vi "PH_gentec_P-Link.set Head Attenuator.vi"(0 "i ref in":refnum<vi>, 2 "VISA resource in":refnum<visa-resource-name>, 5 "error in":errorcluster) -> (11 "Timeout":bool, 13 "Data read":string[](array[string]), 14 "i ref out":refnum<vi>, 16 "VISA resource out":refnum<visa-resource-name>, 17 "Error":bool, 19 "error out":errorcluster)   [LabVIEW 2014, in "PH_gentec_P-Link.lvlib"]
doc: "This VI writes wanted Settings to the Device and checks the result."
uses:
  PH_gentec_P-Link.lvlib
  instr.lib/Gentec-M-Link/gentec-M-Link - Driver.lvlib
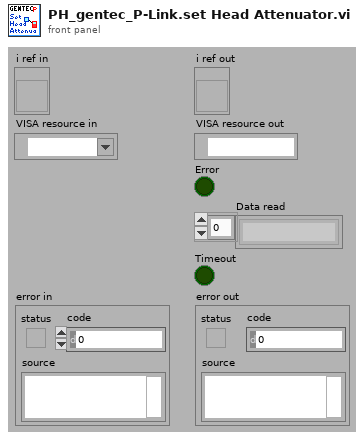
[diagram p1: front panel]
types:
  T1 = typedef "PH_gentec_P-Link.lvlib/PH_gentec_P-Link.i attribute.ctl" = cluster{"GUI References":cluster{"Wanted Head Settings":refnum<vi>, "Current Head Settings":refnum<vi>, "Set Auto Range":refnum<vi>, "Trigger Polarity":refnum<vi>, "Trigger Source":refnum<vi>, "Waveform Averages":refnum<vi>, "Continuous":refnum<vi>, "get one Value":refnum<vi>}, "Wanted Head Settings":T2, "Current Head Settings":T2}
  T2 = typedef "PH_gentec_P-Link.lvlib/PH_gentec_P-Link.Head Settings.ctl" = cluster{"Measurement Mode":T3, "Enable Anticipation":bool, "Set Auto Range":bool, "Block Signal":bool, "Set Head Attenuator":bool, "Enable SSE":bool, "Trigger Polarity":T4, "Trigger Source":T5, "Waveform Averages":T6, "Set Zero":i32, "Current":i32, "Start Data Flow":bool}
  T3 = typedef "gentec-M-Link - Driver.lvlib/gentec-M-Link.Measurement Mode.ctl" = u16
  T4 = typedef "gentec-M-Link - Driver.lvlib/gentec-M-Link.Trigger Polarity.ctl" = u16
  T5 = typedef "gentec-M-Link - Driver.lvlib/gentec-M-Link.Trigger Source.ctl" = u16
  T6 = typedef "gentec-M-Link - Driver.lvlib/gentec-M-Link.Waveform Averages.ctl" = u16
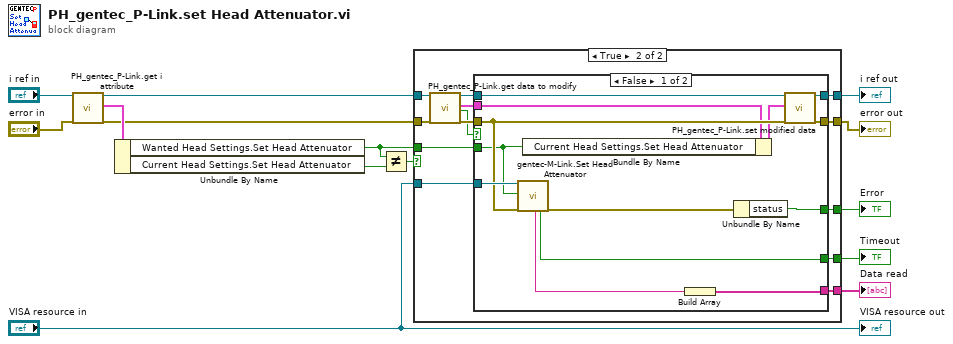
[diagram p0: block diagram]
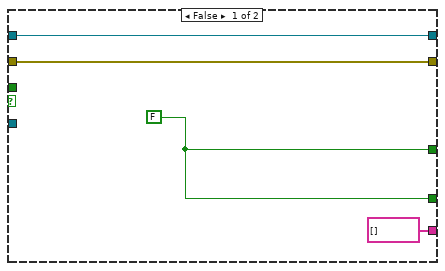
[diagram p2: hidden frame]
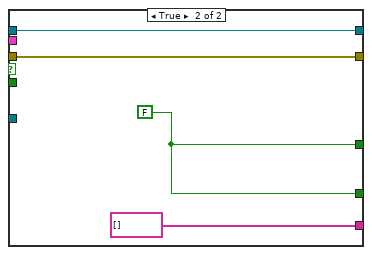
[diagram p3: hidden frame]
diagram:
  n1 = call "PH_gentec_P-Link.get i attribute.vi"("i ref in"="i ref in", "error in (no error)"="error in") -> ("i ref out"=w7:refnum<vi>, "i attribute"=w10:T1, "error out"=w9:errorcluster)  [unwired: 15 in]
  n2 = Unbundle By Name(w10) -> ("Wanted Head Settings.Set Head Attenuator"=w12:bool, "Current Head Settings.Set Head Attenuator"=w11:bool)
  n3 = Not Equal?(x=w12, y=w11) -> (x != y?=w1:bool)
  n4 = case shown="True" w1 {
    tunnel: [w17 w31] -> w14
    tunnel: [w18 w30] -> w13
    tunnel: w12 -> [_ w29]
    tunnel: w9 -> [w17 w24]
    tunnel: w7 -> [w18 w23]
    tunnel: "VISA resource in" -> [_ w22]
    tunnel: [w16 w21] -> w4
    tunnel: [w16 w20] -> w3
    tunnel: [string[] [] w19] -> w2
    frame False {
      w16 = FALSE ("Read Timeout")
    }
    frame True {
      n5 = call "PH_gentec_P-Link.get data to modify.vi"("i ref in"=w23, "error in (no error)"=w24) -> ("i ref out"=w27:refnum<vi>, "i attribute"=w26:T1, "timed out"=w25:bool, "error out"=w28:errorcluster)  [unwired: 14 in]
      n6 = case shown="False" w25 {
        tunnel: w22 -> [w43 _]
        tunnel: [w39 w48] -> w30
        tunnel: [w38 w47] -> w31
        tunnel: w28 -> [w42 w47]
        tunnel: w27 -> [w44 w48]
        tunnel: w26 -> [w41 _]
        tunnel: w29 -> [w40 _]
        tunnel: [w36 w46] -> w21
        tunnel: [w35 w46] -> w20
        tunnel: [w34 string[] []] -> w19
        frame False {
          n7 = call "gentec-M-Link.Set Head Attenuator.vi"("VISA resource In"=w43, "Set Head Attenuator"=w40, "error in (no error)"=w42) -> ("Data Read"=w32:string, "Read Timeout"=w35:bool, "error out"=w33:errorcluster)  [unwired: 11 in, 3 out]
          n8 = Bundle By Name(cluster=w41, "Current Head Settings.Set Head Attenuator"=w40) -> (w37:T1)
          n9 = Build Array(w32) -> (w34:string[])
          n10 = Unbundle By Name(w33) -> ("status"=w36:bool)
          n11 = call "PH_gentec_P-Link.set modified data.vi"("i ref in"=w44, "i attribute"=w37, "error in (no error)"=w42) -> ("i ref out"=w39:refnum<vi>, "error out"=w38:errorcluster)  [unwired: 15 in]
        }
        frame True {
          w46 = FALSE ("Read Timeout")
        }
      }
    }
  }
  "error out" <- w14
  "i ref out" <- w13
  "Error" <- w4
  "Timeout" <- w3
  "Data read" <- w2
  "VISA resource out" <- "VISA resource in"
